vi "JogStepInterpeter (SubVI).vi"(1 "Jog step size ENUM":T2) -> (0 "Jog step size":T1)   [LabVIEW 2016]
uses:
  Enum_TypeDefinitions/Enum_TypeDef_JogStepSize.ctl
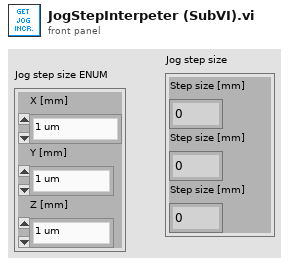
[diagram p1: front panel]
types:
  T1 = cluster{"Step size [mm]":dbl, "Step size [mm]":dbl, "Step size [mm]":dbl}
  T2 = typedef "Enum_TypeDef_JogStepSize.ctl" = cluster{"X [mm]":enum16{"1 um", "5 um", "10 um", "0.1 mm", "0.25 mm", "0.5 mm", "1 mm", "5 mm", "10 mm", "20 mm", "50 mm"}, "Y [mm]":enum16{"1 um", "5 um", "10 um", "0.1 mm", "0.25 mm", "0.5 mm", "1 mm", "5 mm", "10 mm", "20 mm", "50 mm"}, "Z [mm]":enum16{"1 um", "5 um", "10 um", "0.1 mm", "0.25 mm", "0.5 mm", "1 mm", "5 mm", "10 mm", "20 mm", "[None]"}}
  T3 = enum16{"1 um", "5 um", "10 um", "0.1 mm", "0.25 mm", "0.5 mm", "1 mm", "5 mm", "10 mm", "20 mm", "50 mm"}
  T4 = enum16{"1 um", "5 um", "10 um", "0.1 mm", "0.25 mm", "0.5 mm", "1 mm", "5 mm", "10 mm", "20 mm", "[None]"}
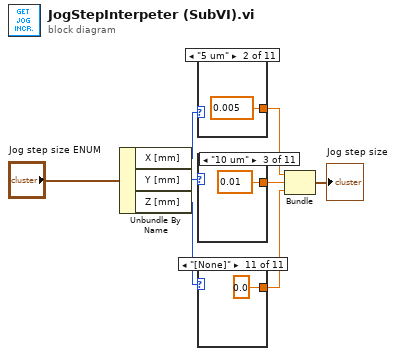
[diagram p0: block diagram]
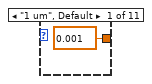
[diagram p2: hidden frame]
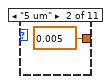
[diagram p3: hidden frame]
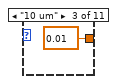
[diagram p4: hidden frame]
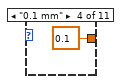
[diagram p5: hidden frame]
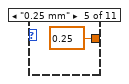
[diagram p6: hidden frame]
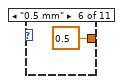
[diagram p7: hidden frame]
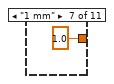
[diagram p8: hidden frame]
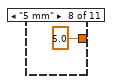
[diagram p9: hidden frame]
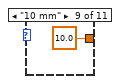
[diagram p10: hidden frame]
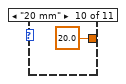
[diagram p11: hidden frame]
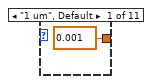
[diagram p12: hidden frame]
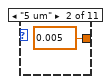
[diagram p13: hidden frame]
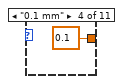
[diagram p14: hidden frame]
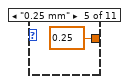
[diagram p15: hidden frame]
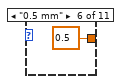
[diagram p16: hidden frame]
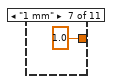
[diagram p17: hidden frame]
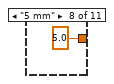
[diagram p18: hidden frame]
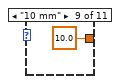
[diagram p19: hidden frame]
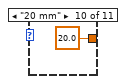
[diagram p20: hidden frame]
diagram:
  n1 = Unbundle By Name("Jog step size ENUM") -> ("X [mm]"=w8:T3, "Y [mm]"=w5:T3, "Z [mm]"=w2:T4)
  n2 = case shown="\"5 um\"" w8 {
    tunnel: [0.001 ("Step size [mm]") 0.005 ("Step size [mm]") 0.01 ("Step size [mm]") 0.1 ("Step size [mm]") 0.25 ("Step size [mm]") 0.5 ("Step size [mm]") 1.0 ("Step size [mm]") 5.0 ("Step size [mm]") 10.0 ("Step size [mm]") 20.0 ("Step size [mm]") 50.0 ("Step size [mm]")] -> w7
    frame "1 um", Default {
    }
    frame "5 um" {
    }
    frame "10 um" {
    }
    frame "0.1 mm" {
    }
    frame "0.25 mm" {
    }
    frame "0.5 mm" {
    }
    frame "1 mm" {
    }
    frame "5 mm" {
    }
    frame "10 mm" {
    }
    frame "20 mm" {
    }
    frame "50 mm" {
    }
  }
  n3 = case shown="\"10 um\"" w5 {
    tunnel: [0.001 ("Step size [mm]") 0.005 ("Step size [mm]") 0.01 ("Step size [mm]") 0.1 ("Step size [mm]") 0.25 ("Step size [mm]") 0.5 ("Step size [mm]") 1.0 ("Step size [mm]") 5.0 ("Step size [mm]") 10.0 ("Step size [mm]") 20.0 ("Step size [mm]") 50.0 ("Step size [mm]")] -> w6
    frame "1 um", Default {
    }
    frame "5 um" {
    }
    frame "10 um" {
    }
    frame "0.1 mm" {
    }
    frame "0.25 mm" {
    }
    frame "0.5 mm" {
    }
    frame "1 mm" {
    }
    frame "5 mm" {
    }
    frame "10 mm" {
    }
    frame "20 mm" {
    }
    frame "50 mm" {
    }
  }
  n4 = case shown="\"[None]\"" w2 {
    tunnel: [0.001 ("Step size [mm]") 0.005 ("Step size [mm]") 0.01 ("Step size [mm]") 0.1 ("Step size [mm]") 0.25 ("Step size [mm]") 0.5 ("Step size [mm]") 1.0 ("Step size [mm]") 5.0 ("Step size [mm]") 10.0 ("Step size [mm]") 20.0 ("Step size [mm]") 0.0 ("Step size [mm]")] -> w1
    frame "1 um", Default {
    }
    frame "5 um" {
    }
    frame "10 um" {
    }
    frame "0.1 mm" {
    }
    frame "0.25 mm" {
    }
    frame "0.5 mm" {
    }
    frame "1 mm" {
    }
    frame "5 mm" {
    }
    frame "10 mm" {
    }
    frame "20 mm" {
    }
    frame "[None]" {
    }
  }
  n5 = Bundle("Step size [mm]"=w7, "Step size [mm]"=w6, "Step size [mm]"=w1) -> (→"Jog step size":T1)  [unwired: 1 in]
